vi "oa_Demodulation Initial States (1 Channel).vi"(4 "filters":T1[](array[typedef]) {"coefficients" format="%.2f"}, 6 "CIC filter settings":T2={"interpolation/decimation factor"=2, "stages"=2, "lag"=1}, 7 "reset? (F)":bool, 9 "imaginary state in":cluster{cluster{dbl[]}, cluster{dbl[]}[]}, 10 "real state in":cluster{cluster{dbl[]}, cluster{dbl[]}[]}, 11 "phase in":dbl format="%.2f") -> (1 "imaginary state out":cluster{cluster{dbl[]}, cluster{dbl[]}[]}, 2 "real state out":cluster{cluster{dbl[]}, cluster{dbl[]}[]}, 3 "phase out":dbl format="%.2f")   [LabVIEW 2017, in "SoundVib_FaultAnalysis.lvlib"]
uses:
  <vilib>/addons/Sound and Vibration/Order Analysis/Fault Analysis/SoundVib_FaultAnalysis.lvlib
  <vilib>/addons/_NISVFA/_Shared subVIs/Controls/OAT Decimation Filter.ctl
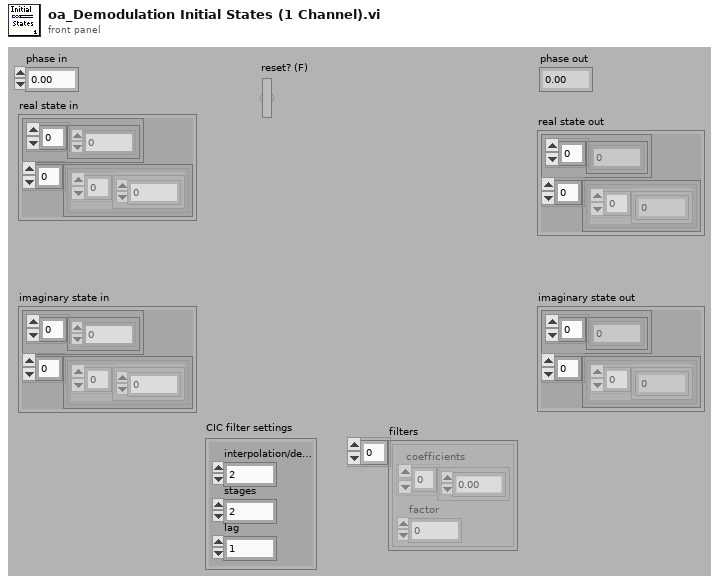
[diagram p1: front panel]
types:
  T1 = typedef "OAT Decimation Filter.ctl" = cluster{"coefficients":dbl[], "factor":i32}
  T2 = cluster{"interpolation/decimation factor":i32, "stages":i32, "lag":i32}
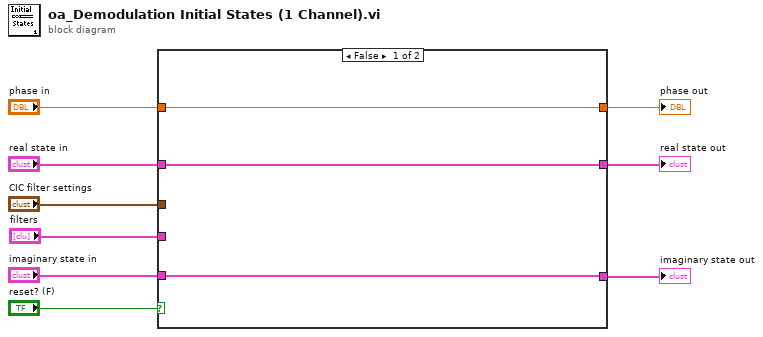
[diagram p0: block diagram]
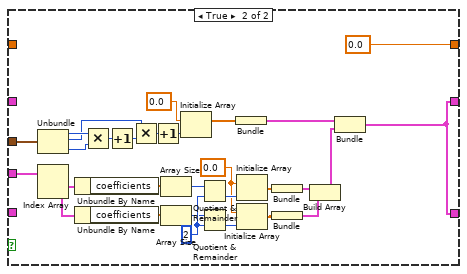
[diagram p2: hidden frame]
diagram:
  n1 = case shown="False" "reset? (F)" {
    tunnel: "real state in" -> [w11 _]
    tunnel: "imaginary state in" -> [w10 _]
    tunnel: [w12 0.0 ("Element Data")] -> w8
    tunnel: "phase in" -> [w12 _]
    tunnel: "CIC filter settings" -> [_ w41]
    tunnel: "filters" -> [_ w40]
    tunnel: [w11 w13] -> w3
    tunnel: [w10 w13] -> w2
    frame False {
    }
    frame True {
      w21 = 0.0 ("Element Data")
      w26 = 2 ("Element Data")
      n2 = Unbundle(w41) -> ("interpolation/decimation factor"=w37:i32, "stages"=w33:i32, "lag"=w36:i32)
      n3 = Index Array(array=w40) -> (element #1=w30:T1, element #2=w29:T1)  [unwired: 2 in]
      n4 = Unbundle By Name(w30) -> ("coefficients"=w28:dbl[])
      n5 = Unbundle By Name(w29) -> ("coefficients"=w27:dbl[])
      n6 = Multiply(x=w37, y=w36) -> (x*y=w35:i32)
      n7 = Increment(x=w35) -> (x+1=w34:i32)
      n8 = Multiply(x=w33, y=w34) -> (x*y=w32:i32)
      n9 = Increment(x=w32) -> (x+1=w31:i32)
      n10 = Array Size(array=w28) -> (size(s)=w25:i32)
      n11 = Array Size(array=w27) -> (size(s)=w24:i32)
      n12 = Initialize Array(0.0 ("Element Data"), w31) -> (w38:dbl[])
      n13 = Quotient & Remainder(x=w25, y=w26) -> (floor(x/y)=w23:i32)  [unwired: 1 out]
      n14 = Quotient & Remainder(x=w24, y=w26) -> (floor(x/y)=w22:i32)  [unwired: 1 out]
      n15 = Bundle(w38) -> (w18:cluster{dbl[]})  [unwired: 1 in]
      n16 = Initialize Array(w21, w23) -> (w19:dbl[])
      n17 = Initialize Array(w21, w22) -> (w20:dbl[])
      n18 = Bundle(w19) -> (w17:cluster{dbl[]})  [unwired: 1 in]
      n19 = Bundle(w20) -> (w16:cluster{dbl[]})  [unwired: 1 in]
      n20 = Build Array(w17, w16) -> (w15:cluster{dbl[]}[])
      n21 = Bundle(w18, w15) -> (w13:cluster{cluster{dbl[]}, cluster{dbl[]}[]})  [unwired: 1 in]
    }
  }
  "phase out" <- w8
  "real state out" <- w3
  "imaginary state out" <- w2
